vi "Reset Symbols.vi"(8 "error in (no error)":errorcluster, 11 "ResultTree in":refnum<class "ResultTree.lvclass">) -> (0 "error out":errorcluster, 3 "ResultTree out":refnum<class "ResultTree.lvclass">)   [LabVIEW 2017, in "ResultTree.lvclass"]
uses:
  ResultTree.lvclass
  Test Outcome.ctl
  ResultTree.lvclass/ResultTree.ctl
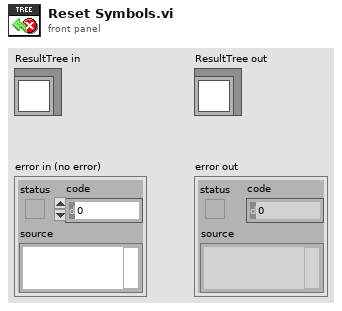
[diagram p1: front panel]
types:
  T1 = typedef "Test Outcome.ctl" = enum16{"None", "Passed", "Failed"}
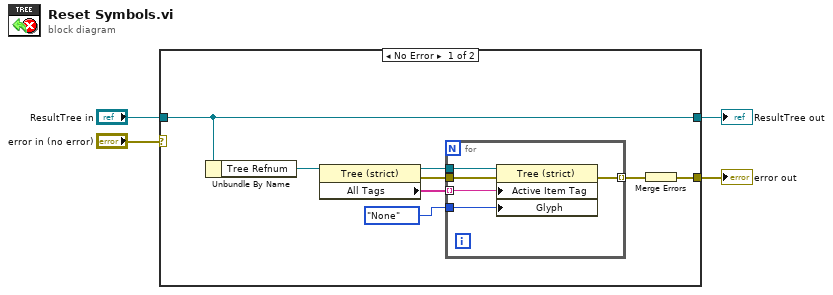
[diagram p0: block diagram]
diagram:
  n1 = case shown="No Error" "error in (no error)" {
    selector: "error in (no error)" -> [_ w19]
    tunnel: [w10 w19] -> w3
    tunnel: [w8 w18] -> w1
    tunnel: "ResultTree in" -> [w8 w18]
    frame No Error {
      n2 = Unbundle By Name(w8) -> ("Tree Refnum"=w5:refnum<vi>)
      n3 = property class="Tree (strict)"(reference=w5) -> (reference out=w9:refnum<vi>, error out=w6:errorcluster, "All Tags"=w11:string[])  [unwired: 1 in]
      n4 = for {
        tunnel: Test_Outcome."None" ("Test Outcome") -> [w16]
        tunnel: w11 -> [w17] mode=indexing
        tunnel: w9 -> [w15]
        tunnel: [w14] -> w7 mode=indexing
        tunnel: w6 -> [w13]
        n5 = property class="Tree (strict)"(reference=w15, error in=w13, "Active Item Tag"=w17, "Glyph"=w16) -> (error out=w14:errorcluster)  [unwired: 1 out]
      }
      n6 = Merge Errors(w7) -> (w10:errorcluster)
    }
    frame Error {
    }
  }
  "error out" <- w3
  "ResultTree out" <- w1
